vi "PH_PSDBController.evt call set Shotcomment.vi"(0 "i ref in":refnum<vi>, 2 "Instance":string, 3 "Shot Comment":string, 5 "error in (no error)":errorcluster) -> (14 "i ref out":refnum<vi>, 19 "error out":errorcluster)   [LabVIEW 2014, in "PH_PSDBController.lvlib"]
doc: "This VI calls the case \"SetShotComment\" by a simple call."
uses:
  PH_PSDBController.lvlib
  CSCore/CSSystem/CoreLib/CoreLib.string 2 byte array.vi
  CSCore/BaseProcess/BaseProcess.lvlib
  CSCore/CSSystem/CoreLib/CoreLib.lvlib
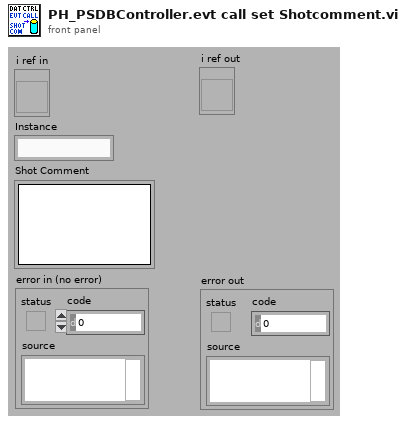
[diagram p1: front panel]
types:
  T1 = typedef "CoreDefs.rawDataType.ctl" = i8[]
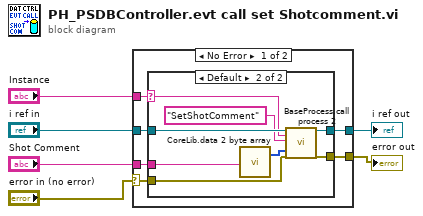
[diagram p0: block diagram]
diagram:
  n1 = case shown="No Error" "error in (no error)" {
    selector: "error in (no error)" -> [w8 w23]
    tunnel: [w12 w24] -> w3
    tunnel: [w11 w23] -> w2
    tunnel: "i ref in" -> [w10 w24]
    tunnel: "Instance" -> [w9 _]
    tunnel: "Shot Comment" -> [w7 _]
    frame No Error {
      n2 = case shown="Default" w9 {
        selector: w9 -> [_ w18]
        tunnel: [w14 w22] -> w12
        tunnel: [w13 w21] -> w11
        tunnel: w10 -> [w14 w20]
        tunnel: w8 -> [w13 w15]
        tunnel: w7 -> [_ w16]
        frame "N/A" {
        }
        frame Default {
          n3 = call-poly "CoreLib.data 2 byte array.vi"("string"=w16) -> ("byteArray out"=w17:T1)  [unwired: 18 in]
          n4 = call "BaseProcess.call process 2.vi"("i ref in"=w20, "Object"=w18, "Selector"="SetShotComment", "Data"=w17, "error in (no error)"=w15) -> ("i ref out"=w22:refnum<vi>, "error out"=w21:errorcluster)  [unwired: 13 in]
        }
      }
    }
    frame Error {
    }
  }
  "error out" <- w2
  "i ref out" <- w3
